vi "Collector Lift LUT.vi"(11 "Collector Lift State":T1) -> (3 "Collector Lift Setpoint":dbl)   [LabVIEW 2015]
uses:
  Typedefs/CollectorLiftStates.ctl
  Gensubs/Bert_or_Ernie.vi
panel:
  in  "Pratice Bot Collector Lift LUT":dbl[](array[numeric])
  in  "Comp Bot Collector Lift LUT":dbl[](array[numeric])
  # "C. Manual"
  # "Stow"
  # "Collect Position"
  # "Spit Position"
  # "PC Set Up"
  # "PC Lift Up"
  # "CDF Set Up"
  # "Push CDF Down"
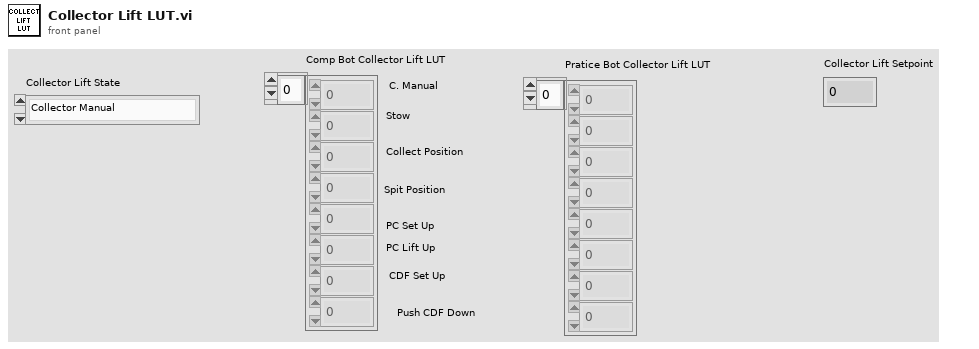
[diagram p1: front panel]
types:
  T1 = typedef "CollectorLiftStates.ctl" = enum16{"Collector Manual", "Stow", "Collect Position", "Spit Position", "Portcullis Set Up", "Portcullis Lift Up", "CDF Set Up", "Push CDF Down"}
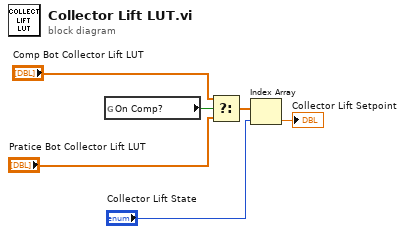
[diagram p0: block diagram]
diagram:
  n1 = global read "Bert_or_Ernie.vi" "On Comp?"() -> (w6:bool)
  n2 = Select(t="Comp Bot Collector Lift LUT", s=w6, f="Pratice Bot Collector Lift LUT") -> (s? t:f=w2:dbl[])
  n3 = Index Array(array=w2, index="Collector Lift State") -> (element=→"Collector Lift Setpoint":dbl)
